vi "IdentityCheck.vi"(8 "error in (no error)":errorcluster, 11 "EMTestCWS500N in":refnum<class "EMTestCWS500N.lvclass">) -> (0 "error out":errorcluster, 3 "EMTestCWS500N out":refnum<class "EMTestCWS500N.lvclass">)   [LabVIEW 2013, in "EMTestCWS500N.lvclass"]
uses:
  EMTestCWS500N.lvclass
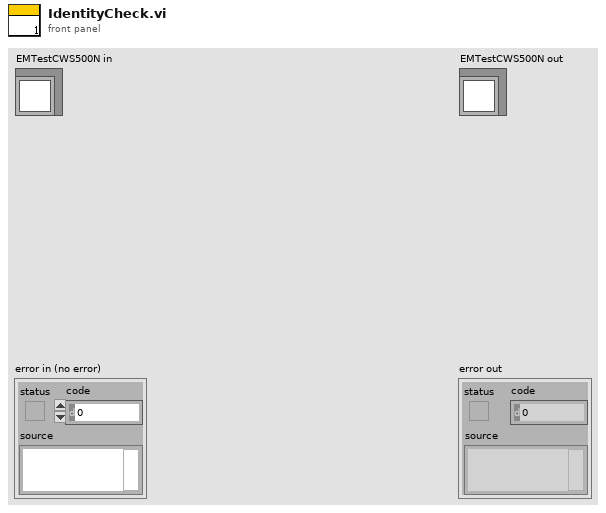
[diagram p1: front panel]
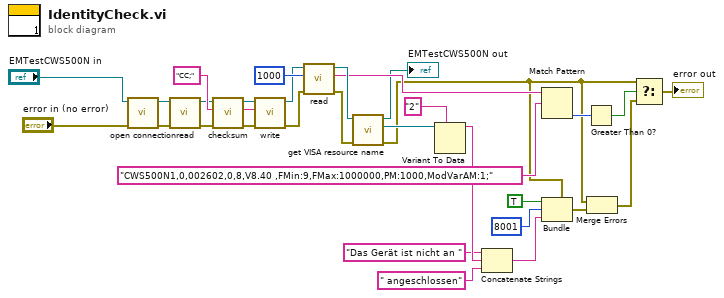
[diagram p0: block diagram]
diagram:
  n1 = call-dynamic "open connection.vi"("error in (no error)"="error in (no error)", "EMTestCWS500N in"="EMTestCWS500N in") -> ("error out"=w3:errorcluster, "EMTestCWS500N out"=w4:refnum<class "EMTestCWS500N.lvclass">)  [unwired: 8 in]
  n2 = call-dynamic "read.vi"("error in (no error)"=w3, "EMTestCWS500N in"=w4) -> ("error out"=w1:errorcluster, "EMTestCWS500N out"=w2:refnum<class "EMTestCWS500N.lvclass">)  [unwired: 7 in, 1 out]
  n3 = call-dynamic "checksum.vi"("error in (no error)"=w1, "input"="CC;", "EMTestCWS500N in"=w2) -> ("error out"=w11:errorcluster, "output"=w14:string, "EMTestCWS500N out"=w12:refnum<class "EMTestCWS500N.lvclass">)  [unwired: 6 in]
  n4 = call-dynamic "write.vi"("error in (no error)"=w11, "String to send"=w14, "EMTestCWS500N in"=w12) -> ("error out"=w16:errorcluster, "EMTestCWS500N out"=w15:refnum<class "EMTestCWS500N.lvclass">)  [unwired: 7 in]
  n5 = call-dynamic "read.vi"("error in (no error)"=w16, "timeout (ms)"=1000, "EMTestCWS500N in"=w15) -> ("error out"=w7:errorcluster, "Return String"=w18:string, "EMTestCWS500N out"=w22:refnum<class "EMTestCWS500N.lvclass">)  [unwired: 6 in]
  n6 = call-dynamic "get VISA resource name.vi"("error in (no error)"=w7, "DeviceInterface (Eingang)"=w22) -> ("error out"=w6:errorcluster, "VISA resource name"=w23:refnum<visa-resource-name>, "DeviceInterface (Ausgang)"=→"EMTestCWS500N out":refnum<class "EMTestCWS500N.lvclass">)  [unwired: 7 in]
  n7 = Variant To Data(type="2" ("input"), Variant=w23) -> (data=w28:string)  [unwired: 1 in, 1 out]
  n8 = Concatenate Strings("Das Gerät ist nicht an " ("string"), w28, " angeschlossen" ("string")) -> (w30:string)
  n9 = Match Pattern(string=w18, regular expression="CWS500N1,0,002602,0,8,V8.40 ,FMin:9,FMax:1000000,PM:1000,ModVarAM:1;") -> (offset past match=w20:i32)  [unwired: 1 in, 3 out]
  n10 = Bundle(cluster=w6, "status"=TRUE, "code"=8001, "source"=w30) -> (w31:errorcluster)
  n11 = Greater Than 0?(x=w20) -> (x > 0?=w21:bool)
  n12 = Merge Errors(w6, w31) -> (w32:errorcluster)
  n13 = Select(t=w6, s=w21, f=w32) -> (s? t:f=→"error out":errorcluster)
